vi "udp parameters9.vi"() -> (0 "Active Timeout UDP Read 2":bool, 3 "Timeout UDP Read ms 2":i32, 4 "Receive Buffer Size 2":u32, 5 "Max Bytes/Read  2":i32, 6 "Port 2":i32)   [LabVIEW 2011]
panel:
  in  "stop":bool
  in  "OK Button":bool
  in  "Active Timeout UDP Read":bool
  in  "Timeout UDP Read ms":i32
  in  "Receive Buffer Size":u32
  in  "Max Bytes/Read":i32
  in  "Port":i32
  # "UDP TRANSFER CONDITIONS"
  # "ON"
  # "OFF"
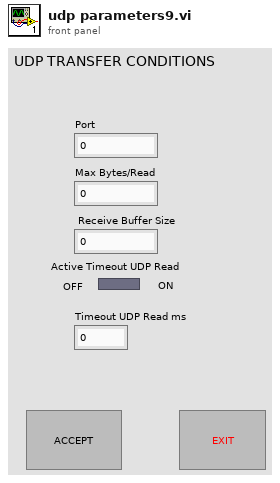
[diagram p1: front panel]
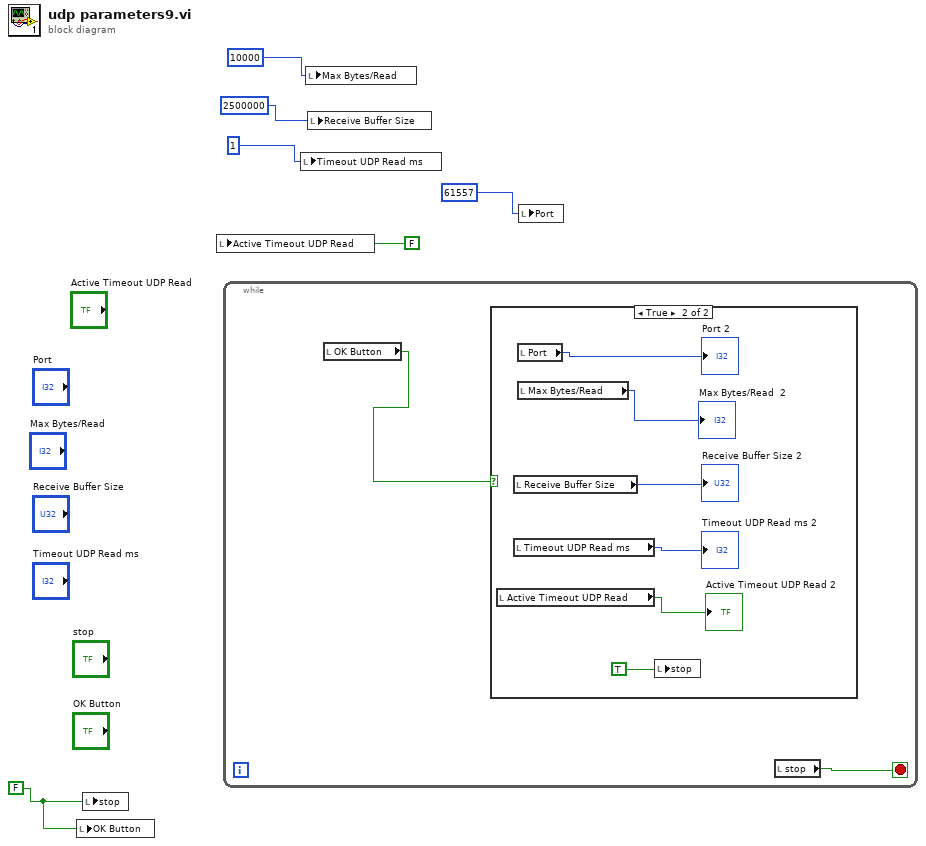
[diagram p0: block diagram]
diagram:
  w6 = FALSE
  n1 = local write "OK Button"(w6) -> ()
  n2 = local write "stop"(w6) -> ()
  n3 = local write "Active Timeout UDP Read"(FALSE) -> ()
  n4 = while {
    stop <- w8 stop-if-true
    n5 = local read "OK Button"() -> (w7:bool)
    n6 = case shown="True" w7 {
      frame False {
      }
      frame True {
        n7 = local read "Active Timeout UDP Read"() -> (→"Active Timeout UDP Read 2":bool)
        n8 = local read "Receive Buffer Size"() -> (→"Receive Buffer Size 2":u32)
        n9 = local read "Timeout UDP Read ms"() -> (→"Timeout UDP Read ms 2":i32)
        n10 = local read "Port"() -> (→"Port 2":i32)
        n11 = local read "Max Bytes/Read"() -> (→"Max Bytes/Read  2":i32)
        n12 = local write "stop"(TRUE) -> ()
      }
    }
    n13 = local read "stop"() -> (w8:bool)
  }
  n14 = local write "Timeout UDP Read ms"(1) -> ()
  n15 = local write "Max Bytes/Read"(10000) -> ()
  n16 = local write "Receive Buffer Size"(u32 2500000) -> ()
  n17 = local write "Port"(61557) -> ()
